vi "ADD USER TO PGSQL.vi"(8 "Image In":T1, 9 "REFERENCES":T3, 10 "USER INFO IN":T4) -> (1 "USER/ITEM DATA TRANSFER":T2(array[cluster]), 2 "USER INFO OUT":T4)   [LabVIEW 2019]
uses:
  Controls/References Cluster.ctl
  <vilib>/userDefined/High Color/IMAQdx.ctl
  Controls/Custom Calendar/Custom Calendar.xctl
  <vilib>/vision/Image Controls.llb/IMAQ Image.ctl
  Controls/Table Data Types/User Data Type.ctl
  <vilib>/addons/database/Connection.llb/DB Tools Open Connec (String).vi
  <vilib>/addons/database/NI_Database_API.lvlib
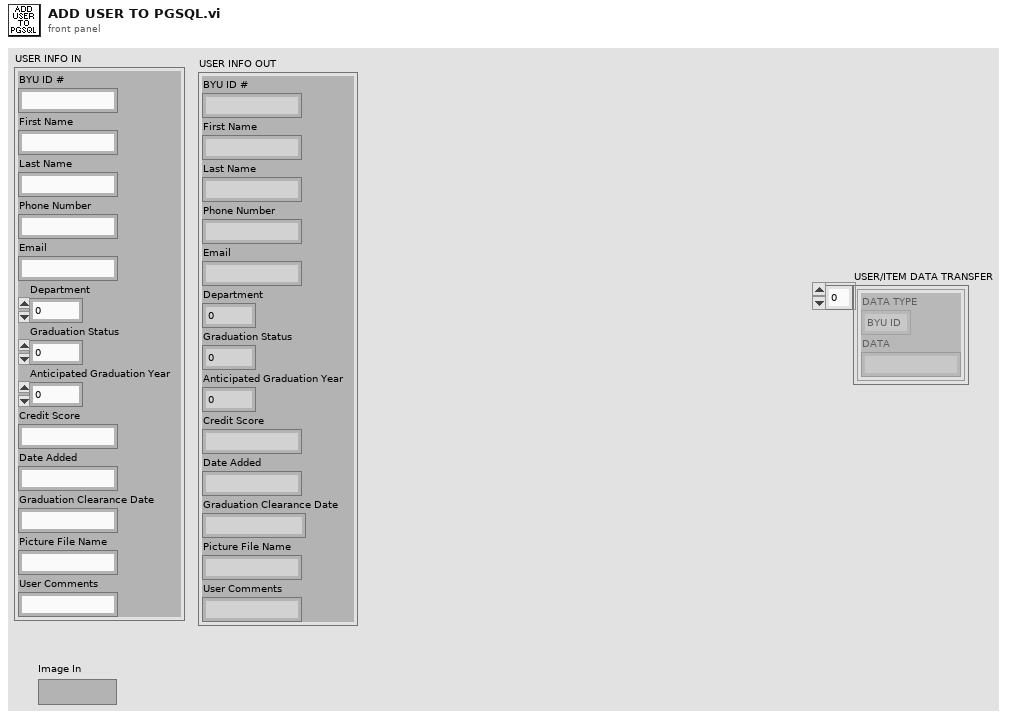
[diagram p1: front panel]
types:
  T1 = typedef "IMAQ Image.ctl" = refnum<image>
  T2 = cluster{"DATA TYPE":enum16{"BYU ID", "ME#/IDENTIFIER", "BYU ICN"}, "DATA":string}[]
  T3 = typedef "References Cluster.ctl" = cluster{"MAIN PAGES":refnum<vi>, "ADD/EDIT ITEM REFERENCES":cluster{"Identifier":refnum<vi>, "BYU ICN #":refnum<vi>, "Item Description":refnum<vi>, "Comments":refnum<vi>, "Checked Out Date":refnum<vi>, "Due Date":refnum<vi>, "Check Out Location":refnum<vi>, "Reminder Count":refnum<vi>, "Most Recent Reminder Date":refnum<vi>, "BYU ID #":refnum<vi>, "Building/Room":refnum<vi>, "Location in Room":refnum<vi>, "Manual":refnum<vi>, "Manufacturer":refnum<vi>, "Model #":refnum<vi>, "Serial #":refnum<vi>, "Date Acquired":refnum<vi>, "ADD/EDIT ITEM LABEL":refnum<vi>, "ARCHIVE ITEM":refnum<vi>, "Archive Item Inputs":refnum<vi>, "Reminder Notes":refnum<vi>, "DUPLICATE ITEM":refnum<vi>}, "ADD/EDIT USER REFERENCES":cluster{"BYU ID # (##-###-####)":refnum<vi>, "First Name":refnum<vi>, "Last Name":refnum<vi>, "Phone Number (###-###-####)":refnum<vi>, "Email":refnum<vi>, "Department":refnum<vi>, "Graduation Status":refnum<vi>, "Anticipated Graduation Year":refnum<vi>, "Credit Score":refnum<vi>, "Date Added":refnum<vi>, "Graduation Clearance Date":refnum<vi>, "Picture File Name":refnum<vi>, "ADD/EDIT USER LABEL":refnum<vi>, "Department Map":refnum<vi>, "Status Map":refnum<vi>, "Anticipated Graduation Year Map":refnum<vi>, "User Agreement":refnum<vi>, "User Comments":refnum<vi>, "Camera":refnum<vi>}, "RETURN ITEM REFERENCES":cluster{"Item or Person:":refnum<vi>, "Search Return Results":refnum<vi>, "What are you searching for?":refnum<vi>}, "SEARCH DATABASE REFERENCES":cluster{"What to Search For:":refnum<vi>, "Where to Search":refnum<vi>, "Column to Search In":refnum<vi>, "Column to Sort By":refnum<vi>, "Search Database Results":refnum<vi>, "Inventory Column Selector":refnum<vi>, "User Column Selector":refnum<vi>, "Inventory Archive Column Selector":refnum<vi>, "User Archive Column Selector":refnum<vi>, "Sales Tracking Column Selector":refnum<vi>, "Checked In Archive Column Selector":refnum<vi>, "Restore User":refnum<vi>, "Date Range":refnum<vi>, "Dates Less Than":refnum<vi>, "Dates Greater Than":refnum<vi>, "Search Print Receipt":refnum<vi>, "Edit Sale Description":refnum<vi>}, "USER ITEMS REFERENCES":cluster{"USER'S INFORMATION":refnum<vi>, "User's Checked Out Items":refnum<vi>, "User Info Comments":refnum<vi>, "SEE USER INFO COMMENTS":refnum<vi>}, "EDIT ITEMS REFERENCES":cluster{"New Check Out Location":refnum<vi>, "Items to Edit":refnum<vi>, "Edit Items Due Date":refnum<vi>, "New Reminder Notes":refnum<vi>, "New Item Description":refnum<vi>}, "CHECK OUT ITEMS REFERENCES":cluster{"Enter Item:":refnum<vi>, "Check Out Items Due Date":refnum<vi>, "Check Out Location":refnum<vi>, "Items to be Checked Out":refnum<vi>, "Possible Items":refnum<vi>, "Altered Item Description":refnum<vi>}, "TRANSFER ITEMS REFERENCES":cluster{"Search Parameter":refnum<vi>, "What to Match":refnum<vi>, "Matching Individuals":refnum<vi>, "Items to be Transferred":refnum<vi>}, "SETTINGS REFERENCES":cluster{"PSC Database Settings":refnum<vi>, "PSC Sales Item Spreadsheet":refnum<vi>}, "PSC SALES REFERENCES":cluster{"BYU ID CARD #":refnum<vi>, "Sale Description":refnum<vi>, "Scan or Enter Item Name":refnum<vi>, "Items to be Sold":refnum<vi>, "Grand Total":refnum<vi>, "Item List":refnum<vi>}}
  T4 = cluster{"BYU ID #":string, "First Name":string, "Last Name":string, "Phone Number":string, "Email":string, "Department":u16, "Graduation Status":u16, "Anticipated Graduation Year":u16, "Credit Score":string, "Date Added":string, "Graduation Clearance Date":string, "Picture File Name":string, "User Comments":string}
  T5 = cluster{"DATA TYPE":enum16{"BYU ID", "ME#/IDENTIFIER", "BYU ICN"}, "DATA":string}
  T6 = typedef "User Data Type.ctl" = cluster{"BYU ID #":string, "First Name":string, "Last Name":string, "Phone Number":string, "Email":string, "Department":string, "Graduation Status":string, "Anticipated Graduation Year":string, "Credit Score":dbl, "Date Added":string, "Graduation Clearance Date":string, "Picture File Name":string, "User Comments":string}
  T7 = cluster{"BYU ID # (##-###-####)":refnum<vi>, "First Name":refnum<vi>, "Last Name":refnum<vi>, "Phone Number (###-###-####)":refnum<vi>, "Email":refnum<vi>, "Department":refnum<vi>, "Graduation Status":refnum<vi>, "Anticipated Graduation Year":refnum<vi>, "Credit Score":refnum<vi>, "Date Added":refnum<vi>, "Graduation Clearance Date":refnum<vi>, "Picture File Name":refnum<vi>, "ADD/EDIT USER LABEL":refnum<vi>, "Department Map":refnum<vi>, "Status Map":refnum<vi>, "Anticipated Graduation Year Map":refnum<vi>, "User Agreement":refnum<vi>, "User Comments":refnum<vi>, "Camera":refnum<vi>}
  T8 = typedef "NI_Database_API.lvlib/Conn ObjectReference.ctl" = refnum<k1>
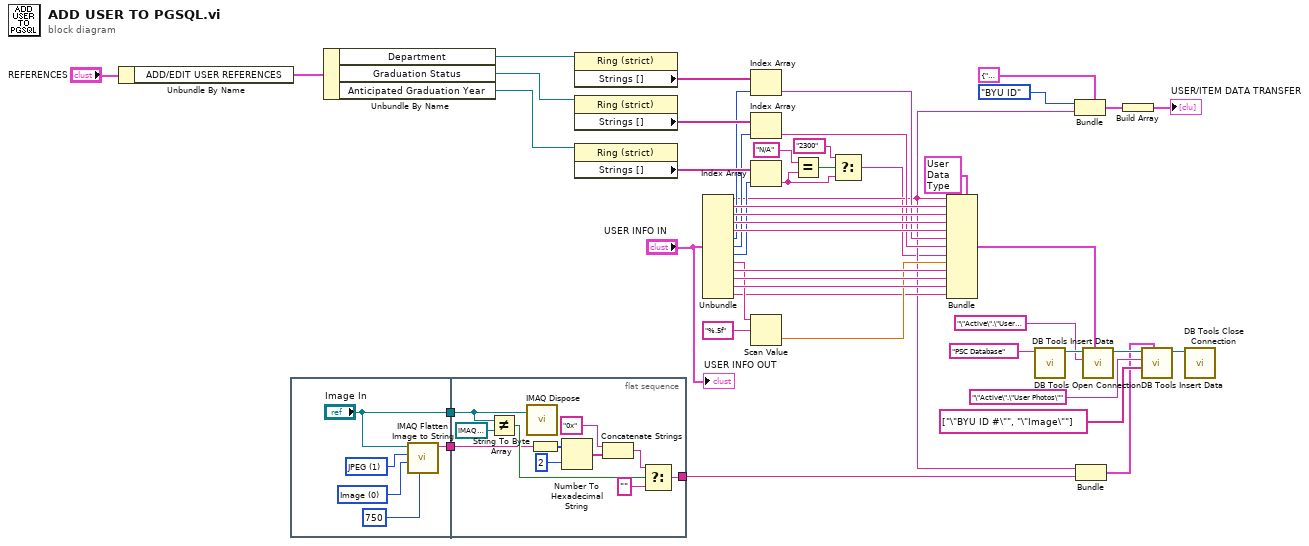
[diagram p0: block diagram]
diagram:
  n1 = Unbundle By Name("REFERENCES") -> ("ADD/EDIT USER REFERENCES"=w38:T7)
  n2 = flat-sequence {
    tunnel: ["Image In"] -> w14
    tunnel: [w49] -> w13
    tunnel: w14 -> [w63]
    tunnel: w13 -> [w56]
    tunnel: [w54] -> w6
    frame #0 {
      w52 = 0 items=["Image", "Image and Vision Info", "Reference to Image"] ("Type of Flatten (Image and Vision Info)")
      w53 = 1 items=["None", "JPEG", "PACKED BINARY"] ("Compression (None)")
      n3 = call "IMAQ Flatten Image to String"("Quality (750)"=750, "Type of Flatten (Image and Vision Info)"=w52, "Compression (None)"=w53, "Image"="Image In") -> ("Data String"=w49:string)  [unwired: 6 in, 1 out]
    }
    frame #1 {
      n4 = Not Equal?(x=w63, y=T1 refnum) -> (x != y?=w62:bool)
      n5 = call "IMAQ Dispose"("Image"=w63) -> ()  [unwired: 5 in, 1 out]
      n6 = String To Byte Array(string=w56) -> (unsigned byte array=w60:u8[])
      n7 = Number To Hexadecimal String(1:i16 2 ("width (-)"), 2:w60) -> (0:w59:string[])
      n8 = Concatenate Strings("0x" ("string"), w59) -> (w55:string)
      n9 = Select(t=w55, s=w62, f="") -> (s? t:f=w54:string)
    }
  }
  n10 = Unbundle By Name(w38) -> ("Department"=w37:refnum<vi>, "Graduation Status"=w36:refnum<vi>, "Anticipated Graduation Year"=w35:refnum<vi>)
  n11 = property class="Ring (strict)"(reference=w37) -> ("Strings []"=w34:string[])  [unwired: 1 in, 2 out]
  n12 = property class="Ring (strict)"(reference=w36) -> ("Strings []"=w33:string[])  [unwired: 1 in, 2 out]
  n13 = property class="Ring (strict)"(reference=w35) -> ("Strings []"=w32:string[])  [unwired: 1 in, 2 out]
  n14 = Unbundle("USER INFO IN") -> ("BYU ID #"=w12:string, "First Name"=w31:string, "Last Name"=w30:string, "Phone Number"=w29:string, "Email"=w28:string, "Department"=w27:u16, "Graduation Status"=w26:u16, "Anticipated Graduation Year"=w25:u16, "Credit Score"=w42:string, "Date Added"=w43:string, "Graduation Clearance Date"=w44:string, "Picture File Name"=w45:string, "User Comments"=w15:string)
  n15 = Index Array(array=w34, index=w27) -> (element=w23:string)
  n16 = Index Array(array=w33, index=w26) -> (element=w24:string)
  n17 = Index Array(array=w32, index=w25) -> (element=w3:string)
  n18 = Scan Value(string=w42, format string="%.5f") -> (value=w40:dbl)  [unwired: 1 in, 1 out]
  n19 = Equal?(x="N/A", y=w3) -> (x = y?=w4:bool)
  n20 = Select(t="2300", s=w4, f=w3) -> (s? t:f=w1:string)
  n21 = Bundle(cluster=T6 {"BYU ID #"="", "First Name"="", "Last Name"="", "Phone Number"="", "Email"="", "Department"="", "Graduation Status"="", "Anticipated Graduation Year"="", "Credit Score"=0.0, "Date Added"="", "Graduation Clearance Date"="", "Picture File Name"="", "User Comments"=""} ("USER DATA TYPE"), "BYU ID #"=w12, "First Name"=w31, "Last Name"=w30, "Phone Number"=w29, "Email"=w28, "Department"=w23, "Graduation Status"=w24, "Anticipated Graduation Year"=w1, "Credit Score"=w40, "Date Added"=w43, "Graduation Clearance Date"=w44, "Picture File Name"=w45, "User Comments"=w15) -> (w22:T6)
  n22 = call-poly <vilib>:"DB Tools Open Connection.vi"("connection information"="PSC Database" ("table")) -> ("connection reference"=w48:T8)  [unwired: 7 in, 1 out]
  n23 = Bundle(cluster=T5 {"DATA TYPE"=enum."BYU ID", "DATA"=""} ("USER/ITEM DATA TRANSFER"), "DATA TYPE"=enum16{"BYU ID", "ME#/IDENTIFIER", "BYU ICN"}."BYU ID", "DATA"=w12) -> (w17:T5)
  n24 = Bundle("BYU ID #"=w12, "f"=w6) -> (w8:cluster{"BYU ID #":string, "f":string})  [unwired: 1 in]
  n25 = call <vilib>:"DB Tools Insert Data.vi"("data"=w22, "table"="\"Active\".\"Users\"", "connection reference"=w48) -> ("connection reference out"=w11:T8)  [unwired: 7 in, 1 out]
  n26 = Build Array(w17) -> (→"USER/ITEM DATA TRANSFER":T2)
  n27 = call <vilib>:"DB Tools Insert Data.vi"("data"=w8, "columns"=string[] ["\"BYU ID #\"", "\"Image\""], "table"="\"Active\".\"User Photos\"", "connection reference"=w11) -> ("connection reference out"=w7:T8)  [unwired: 6 in, 1 out]
  n28 = call <vilib>:"DB Tools Close Connection.vi"("connection reference"=w7) -> ()  [unwired: 6 in, 1 out]
  "USER INFO OUT" <- "USER INFO IN"
